vi "To 1D Bool Tree Data.vi"(10 "1D Bool":bool[](array[boolean])) -> (3 "1D Bool Tree Data":refnum<class "1D Bool.lvclass">)   [LabVIEW 2017, in "Tree API.lvlib" / "1D Bool.lvclass"]
doc: "Convert a 1D Bool value to Tree Data type."
uses:
  1D Bool.lvclass
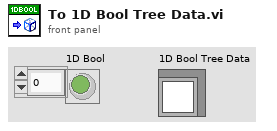
[diagram p1: front panel]
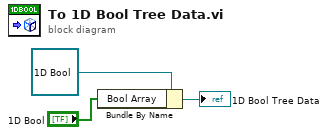
[diagram p0: block diagram]
diagram:
  n1 = Bundle By Name(cluster=refnum<class "1D Bool.lvclass"> refnum ("Bool Array.lvclass"), "Bool Array"="1D Bool") -> (→"1D Bool Tree Data":refnum<class "1D Bool.lvclass">)
